vi "MU Value Of Used Revision.vi"(8 "error in (no error)":errorcluster, 11 "handle":u64) -> (0 "error out (no error)":errorcluster, 2 "revisionId":u32, 3 "function return":u32)   [LabVIEW 2017, in "MU_3SL_interface.lvlib"]
uses:
  MU_3SL_interface.lvlib
  lib/MU_3SL_interface.dll
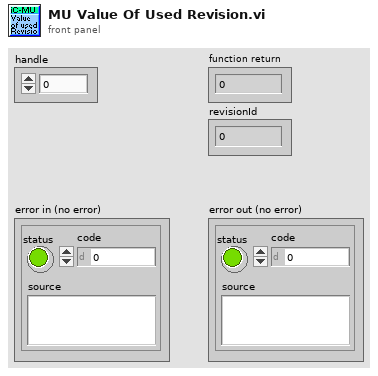
[diagram p1: front panel]
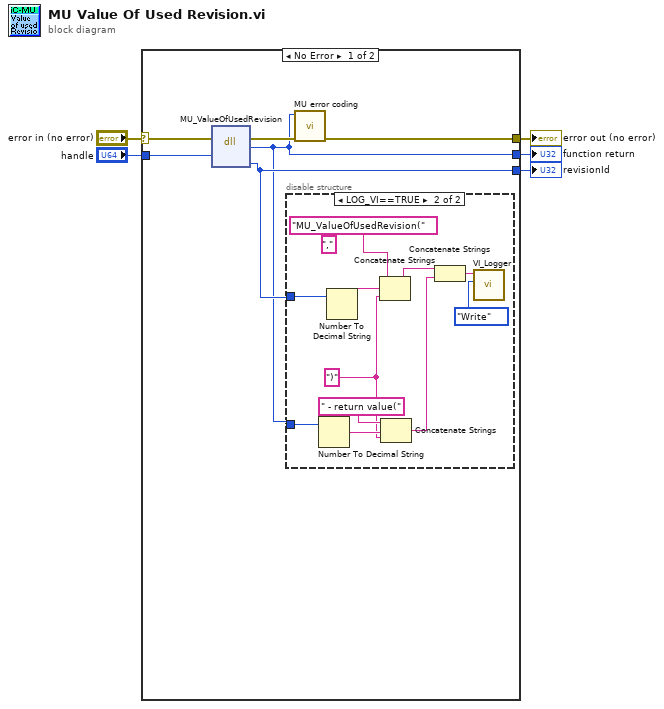
[diagram p0: block diagram]
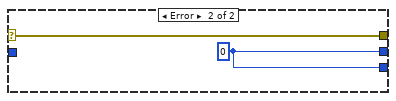
[diagram p3: hidden frame]
diagram:
  n1 = case shown="No Error" "error in (no error)" {
    selector: "error in (no error)" -> [w8 w24]
    tunnel: [w6 w23] -> w5
    tunnel: "handle" -> [w11 _]
    tunnel: [w9 w24] -> w3
    tunnel: [w7 w23] -> w1
    frame No Error {
      n2 = dll-call lib="C:/Users/bes/AppData/Roaming/work/mu_9so/icsubmodules/soft_mu_3sl_master/lv_interface/lib/MU_3SL_interface**.*" fn="MU_ValueOfUsedRevision"(error in=w8, "handle"=w11) -> (error out=w10:errorcluster, "return type"=w6:u32, "revisionId"=w7:u32)  [unwired: 4 in, 1 out]
      n3 = disable-structure shown="LOG_VI==TRUE" {
        disable-tunnel: w6 -> [_ w20]
        disable-tunnel: w7 -> [_ w15]
        frame condition #0 {
        }
        frame condition #1 (active) {
          w12 = ")" ("string")
          (unwired) "," ("string")
          n4 = Number To Decimal String(number=w20) -> (decimal integer string=w19:string)  [unwired: 1 in]
          n5 = Number To Decimal String(number=w15) -> (decimal integer string=w14:string)  [unwired: 1 in]
          n6 = Concatenate Strings("MU_ValueOfUsedRevision(" ("Info in"), w14, w12) -> (w18:string)
          n7 = Concatenate Strings(" - return value(" ("string"), w19, w12) -> (w17:string)
          n8 = Concatenate Strings(w18, w17) -> (w16:string)
          n9 = call "VI_Logger.vi"("Action (Read)"=enum16{"Write", "Read"}."Write", "Info in"=w16) -> ()  [unwired: 8 in, 2 out]
        }
      }
      n10 = call "MU error coding.vi"("error in (no error)"=w10, "function return in"=w6) -> ("error out"=w9:errorcluster)  [unwired: 9 in]
    }
    frame Error {
      w23 = u32 0
    }
  }
  "function return" <- w5
  "error out (no error)" <- w3
  "revisionId" <- w1
